vi "temp.type.vi"(11 "filter.cmd.state.new":cluster{"state":T1, "ob.cmd":T2, "i":i16}={"state"=enum."Wait", "ob.cmd"={"type"=enum."AddOrder", "side"=0, "orderId "=0, "quantity"=0, "symbol"=0, "price"=0, "executed.qty"=0, "canceled.qty"=0, "remaining.qty"=0, "seconds"=0, "nanoseconds"=0, "Add"=FALSE, "Edit"=FALSE, "Remove"=FALSE, "seq no"=0, "recv.time"=0, "parse.time"=0}, "i"=0}) -> ()   [LabVIEW 2020]
uses:
  submodules/Market.Data.Bats.Parser/fpga/poc.ip.debug.states.ctl
  submodules/Market.Data.Common/fpga/orderbook.command.type.ctl
  submodules/Market.Data.Common/fpga/fpganow.common.fpga.lvlib
  submodules/Market.Data.Common/fpga/orderbook.command.ctl
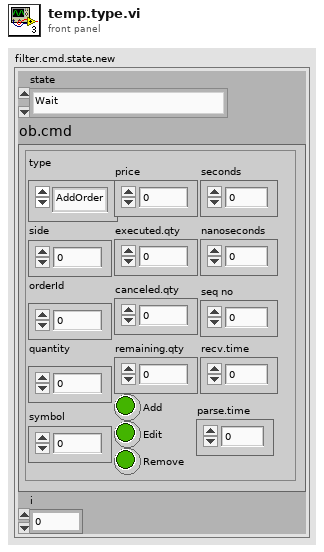
[diagram p1: front panel]
types:
  T1 = typedef "poc.ip.debug.states.ctl" = enum16{"Wait", "Write.Data"}
  T2 = typedef "fpganow.common.fpga.lvlib/orderbook.command.ctl" = cluster{"type":T3, "side":u8, "orderId ":u64, "quantity":u32, "symbol":u64, "price":u64, "executed.qty":u32, "canceled.qty":u32, "remaining.qty":u32, "seconds":u64, "nanoseconds":u64, "Add":bool, "Edit":bool, "Remove":bool, "seq no":u32, "recv.time":u64, "parse.time":u64}
  T3 = typedef "fpganow.common.fpga.lvlib/orderbook.command.type.ctl" = enum8{"Time", "AddOrder", "OrderExecuted", "OrderExecutedAtPrice", "ReduceSize", "ModifyOrder", "DeleteOrder", "Get.Everything", "Get.All.Orders", "Get.Top"}
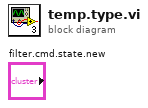
[diagram p0: block diagram]
diagram:
